vi "GFITS_ComposeNextForcedImName.vi"(9 "argument in":string, 11 "Database RefNum in":T1) -> (1 "next fits":string)   [LabVIEW 2016]
uses:
  DBSHAND/private/vis/DatabaseHand_RefNum.ctl
  DBSHAND/private/vis/DatabaseHand_Element_Get(string).vi
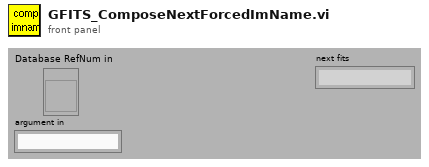
[diagram p1: front panel]
types:
  T1 = typedef "DatabaseHand_RefNum.ctl" = refnum<vi>
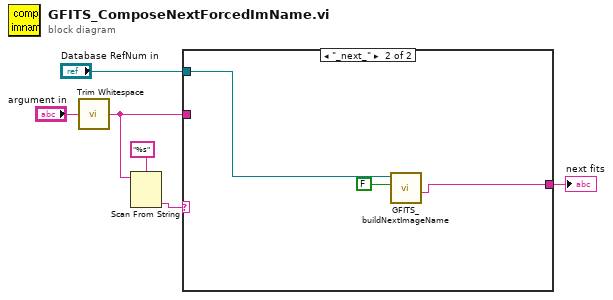
[diagram p0: block diagram]
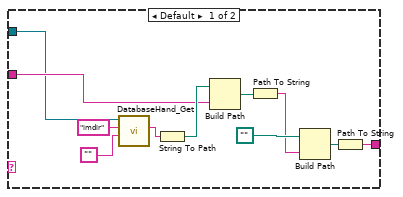
[diagram p2: hidden frame]
diagram:
  n1 = call <vilib>:"Trim Whitespace.vi"("string"="argument in") -> ("trimmed string"=w6:string)  [unwired: 1 in]
  n2 = Scan From String(format string="%s", input string=w6) -> (output 1=w4:string)  [unwired: 2 in, 4 out]
  n3 = case shown="\"_next_\"" w4 {
    tunnel: w6 -> [w11 _]
    tunnel: "Database RefNum in" -> [w10 w20]
    tunnel: [w7 w19] -> w2
    frame Default {
      n4 = call-poly "DatabaseHand_Get.vi"("default value"="", "name"="imdir", "Database RefNum in"=w10) -> ("value"=w15:string)  [unwired: 2 in, 6 out]
      n5 = String To Path(string=w15) -> (path=w14:path)
      n6 = Build Path(base path=w14, name or relative path=w11) -> (appended path=w13:path)
      n7 = Path To String(path=w13) -> (string=w9:string)
      n8 = Build Path(base path=path "", name or relative path=w9) -> (appended path=w8:path)
      n9 = Path To String(path=w8) -> (string=w7:string)
    }
    frame "_next_" {
      n10 = call "GFITS_buildNextImageName.vi"("set dbs"=FALSE, "Database RefNum"=w20) -> ("image path"=w19:string)  [unwired: 2 in, 5 out]
    }
  }
  "next fits" <- w2
